vi "Msg.vi"(7 "jettl in":refnum<class "jettl.lvclass">, 11 "Merge Error Msg Strategy in":refnum<class "Merge Error Msg Strategy.lvclass">) -> (5 "jettl out":refnum<class "jettl.lvclass">)   [LabVIEW 2021, in "jettl Msg Merge Error.lvlib" / "Merge Error Msg Strategy.lvclass"]
uses:
  Merge Error Msg Strategy.lvclass
  jettl/jettl/jettl.lvclass
  jettl Msg Merge Error/jettl Msg Merge Error.lvclass
  Merge Error Msg Strategy.lvclass/Merge Error Msg Strategy.ctl
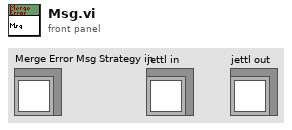
[diagram p1: front panel]
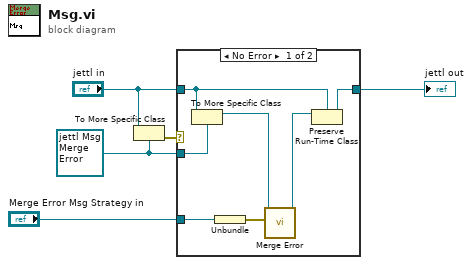
[diagram p0: block diagram]
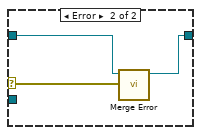
[diagram p2: hidden frame]
diagram:
  w3 = refnum<class "jettl Msg Merge Error.lvclass"> refnum ("jettl.lvlib:Merge Error.lvlib:Merge Error.lvclass")
  n1 = To More Specific Class(target class=w3, reference="jettl in") -> (error out=w5:errorcluster)  [unwired: 1 in, 1 out]
  n2 = case shown="No Error" w5 {
    selector: w5 -> [_ w15]
    tunnel: [w10 w13] -> w1
    tunnel: "jettl in" -> [w11 w14]
    tunnel: w3 -> [w12 _]
    tunnel: "Merge Error Msg Strategy in" -> [w7 _]
    frame No Error {
      n3 = To More Specific Class(target class=w12, reference=w11) -> (specific class reference=w9:refnum<class "jettl Msg Merge Error.lvclass">)  [unwired: 1 in, 1 out]
      n4 = Unbundle(w7) -> (w6:errorcluster)
      n5 = call-dynamic "Merge Error.vi"("Error"=w6, "jettl Msg Merge Error in"=w9) -> ("jettl Msg Merge Error out"=w8:refnum<class "jettl Msg Merge Error.lvclass">)  [unwired: 9 in]
      n6 = Preserve Run-Time Class(object in=w8, 2:w11) -> (object out=w10:refnum<class "jettl.lvclass">)  [unwired: 1 in, 1 out]
    }
    frame Error {
      n7 = call-dynamic "Merge Error.vi"("Error"=w15, "jettl Msg Merge Error in"=w14) -> ("jettl Msg Merge Error out"=w13:refnum<class "jettl.lvclass">)  [unwired: 9 in]
    }
  }
  "jettl out" <- w1
